vi "rqcAlice ServiceNET Read Data (U8).vi"(8 "error in":errorcluster, 11 "rqcAlice ServiceNET in":T1) -> (0 "error out":errorcluster, 1 "data valid":bool, 2 "data":u8[](array[numeric]), 3 "rqcAlice ServiceNET out":T1)   [LabVIEW 2018]
uses:
  Custom Controls/rqcAlice ServiceNET control.ctl
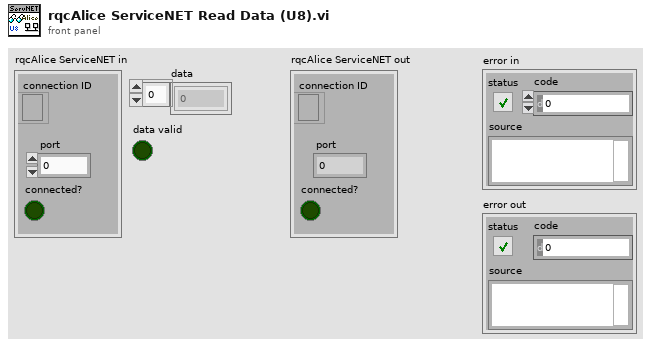
[diagram p1: front panel]
types:
  T1 = typedef "rqcAlice ServiceNET control.ctl" = cluster{"connection ID":refnum<k5>, "port":u16, "connected?":bool}
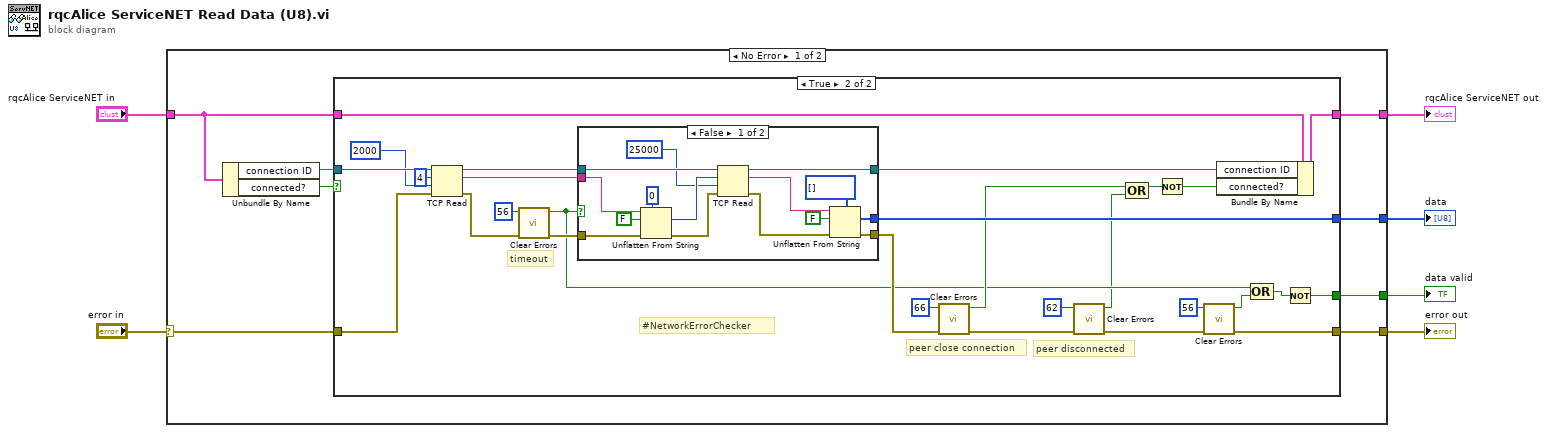
[diagram p0: block diagram]
diagram:
  n1 = case shown="No Error" "error in" {
    selector: "error in" -> [w11 w63]
    tunnel: [w10 w63] -> w5
    tunnel: "rqcAlice ServiceNET in" -> [w12 w62]
    tunnel: [w9 w62] -> w3
    tunnel: [w8 _] -> w2
    tunnel: [w7 _] -> w1
    frame No Error {
      n2 = Unbundle By Name(w12) -> ("connection ID"=w13:refnum<k5>, "connected?"=w14:bool)
      n3 = case shown="True" w14 {
        tunnel: w13 -> [_ w42]
        tunnel: w11 -> [w16 w41]
        tunnel: [w16 w25] -> w10
        tunnel: [w15 w43] -> w9
        tunnel: w12 -> [w15 w44]
        tunnel: [_ w36] -> w8
        tunnel: [_ w30] -> w7
        frame False {
        }
        frame True {
          # "peer disconnected"
          # "timeout"
          # "peer close connection"
          # "#NetworkErrorChecker"
          n4 = TCP Read(connection ID=w42, bytes to read=4, error in (no error)=w41, 9:2000 ("timeout ms (25000)")) -> (connection ID out=w38:refnum<k5>, data out=w39:string, error out=w28:errorcluster)  [unwired: 1 in]
          n5 = call <vilib>:"Clear Errors.vi"("error in (no error)"=w28, "specific error code to clear (0: all)"=56) -> ("error out"=w27:errorcluster, "specific error cleared?"=w22:bool)  [unwired: 4 in]
          n6 = case shown="False" w22 {
            tunnel: w39 -> [w59 _]
            tunnel: w38 -> [w57 w60]
            tunnel: [w56 w60] -> w37
            tunnel: [w49 _] -> w36
            tunnel: [w48 w61] -> w33
            tunnel: w27 -> [w46 w61]
            frame False {
              n7 = Unflatten From String(type=0, binary string=w59, data includes array or string size? (T)=FALSE, error in (no error)=w46) -> (value=w54:i32, error out=w55:errorcluster)  [unwired: 1 in, 1 out]
              n8 = TCP Read(connection ID=w57, bytes to read=w54, error in (no error)=w55, 9:25000 ("timeout ms (25000)")) -> (connection ID out=w56:refnum<k5>, data out=w52:string, error out=w53:errorcluster)  [unwired: 1 in]
              n9 = Unflatten From String(type=u8[] [], binary string=w52, data includes array or string size? (T)=FALSE, error in (no error)=w53) -> (value=w49:u8[], error out=w48:errorcluster)  [unwired: 1 in, 1 out]
            }
            frame True {
            }
          }
          n10 = call <vilib>:"Clear Errors.vi"("error in (no error)"=w33, "specific error code to clear (0: all)"=66) -> ("error out"=w21:errorcluster, "specific error cleared?"=w32:bool)  [unwired: 4 in]
          n11 = call <vilib>:"Clear Errors.vi"("error in (no error)"=w21, "specific error code to clear (0: all)"=62) -> ("error out"=w20:errorcluster, "specific error cleared?"=w18:bool)  [unwired: 4 in]
          n12 = Compound Arithmetic op=OR(w32, w18) -> (w19:bool)
          n13 = Not(x=w19) -> (.not. x?=w31:bool)
          n14 = call <vilib>:"Clear Errors.vi"("error in (no error)"=w20, "specific error code to clear (0: all)"=56) -> ("error out"=w25:errorcluster, "specific error cleared?"=w24:bool)  [unwired: 4 in]
          n15 = Bundle By Name(cluster=w44, "connection ID"=w37, "connected?"=w31) -> (w43:T1)
          n16 = Compound Arithmetic op=OR(w22, w24) -> (w23:bool)
          n17 = Not(x=w23) -> (.not. x?=w30:bool)
        }
      }
    }
    frame Error {
    }
  }
  "rqcAlice ServiceNET out" <- w3
  "error out" <- w5
  "data" <- w2
  "data valid" <- w1
